vi "Asynchronous QMH with Futures - Performance Comparison.vi"() -> ()   [LabVIEW 2017]
uses:
  SubVIs/Command Queue Data.ctl
  Futures/Promise/Promise.lvclass
  Futures/Future/Future.lvclass
panel:
  in  "Wait For Reply (Sync Notifiers)":bool
  out "time taken":dbl
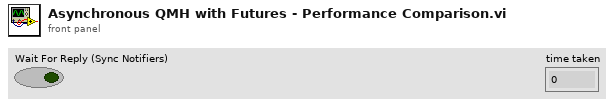
[diagram p1: front panel]
types:
  T1 = typedef "Command Queue Data.ctl" = cluster{"Promise":refnum<class "Promise.lvclass">, "notifier":refnum<notifier>}
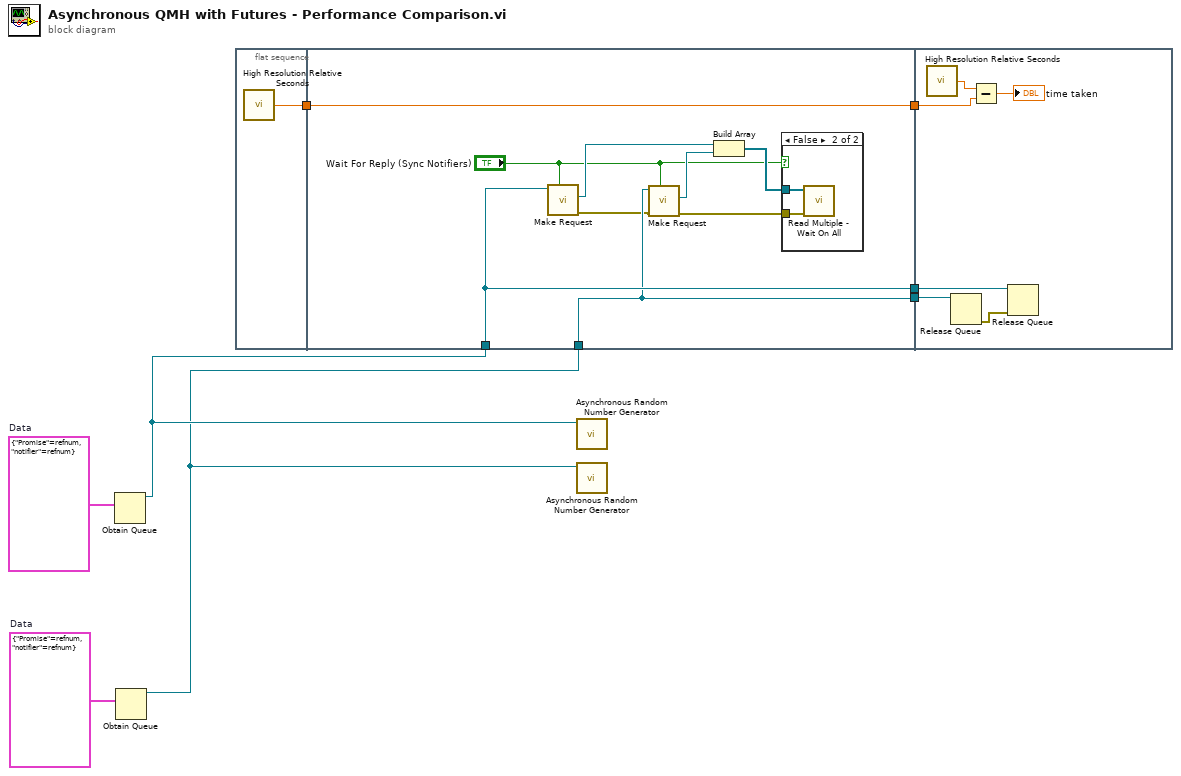
[diagram p0: block diagram]
diagram:
  w7 = T1 {"Promise"=refnum, "notifier"=refnum}  # Data
  w8 = T1 {"Promise"=refnum, "notifier"=refnum}  # Data
  n1 = Obtain Queue(element data type=w8) -> (queue out=w4:refnum<queue>)  [unwired: 4 in, 2 out]
  n2 = Obtain Queue(element data type=w7) -> (queue out=w1:refnum<queue>)  [unwired: 4 in, 2 out]
  n3 = flat-sequence {
    tunnel: [w9] -> w6
    tunnel: w6 -> [w16]
    tunnel: [w16] -> w5
    tunnel: w4 -> [w15]
    tunnel: [w15] -> w3
    tunnel: w1 -> [w14]
    tunnel: [w14] -> w2
    tunnel: w5 -> [w25]
    tunnel: w3 -> [w22]
    tunnel: w2 -> [w21]
    frame #0 {
      n4 = call <vilib>:"High Resolution Relative Seconds.vi"() -> ("relative seconds"=w9:dbl)
    }
    frame #1 {
      n5 = call "Make Request.vi"("Wait For Reply"="Wait For Reply (Sync Notifiers)", "Worker Queue"=w15) -> ("error out"=w12:errorcluster, "Future"=w18:refnum<class "Future.lvclass">)  [unwired: 8 in]
      n6 = call "Make Request.vi"("Wait For Reply"="Wait For Reply (Sync Notifiers)", "error in (no error)"=w12, "Worker Queue"=w14) -> ("error out"=w11:errorcluster, "Future"=w13:refnum<class "Future.lvclass">)  [unwired: 7 in]
      n7 = Build Array(w18, w13) -> (w17:refnum<class "Future.lvclass">[])
      n8 = case shown="False" "Wait For Reply (Sync Notifiers)" {
        tunnel: w17 -> [_ w20]
        tunnel: w11 -> [_ w19]
        frame True {
        }
        frame False {
          n9 = call "Read Multiple - Wait On All.vi"("error in (no error)"=w19, "Futures in"=w20) -> ()  [unwired: 5 in, 5 out]
        }
      }
    }
    frame #2 {
      n10 = call <vilib>:"High Resolution Relative Seconds.vi"() -> ("relative seconds"=w26:dbl)
      n11 = Release Queue(queue=w21) -> (error out=w23:errorcluster)  [unwired: 2 in, 2 out]
      n12 = Subtract(x=w26, y=w25) -> (x-y=→"time taken":dbl)
      n13 = Release Queue(queue=w22, error in (no error)=w23) -> ()  [unwired: 1 in, 3 out]
    }
  }
  n14 = call "Asynchronous Random Number Generator.vi"("Queue in"=w4) -> ()  [unwired: 11 in]
  n15 = call "Asynchronous Random Number Generator.vi"("Queue in"=w1) -> ()  [unwired: 11 in]
